vi "Handle Errors.vi"(8 "error in (no error)":errorcluster, 10 "Location":string, 11 "Mock Error Handler In":refnum<class "Mock Error Handler.lvclass">) -> (0 "error out":errorcluster, 3 "Mock Error Handler Out":refnum<class "Mock Error Handler.lvclass">)   [LabVIEW 2020, in "Mock Error Handler.lvclass"]
uses:
  Mock Error Handler.lvclass
  Mock Error Handler.lvclass/Mock Error Handler.ctl
  Private/Error Message Data.ctl
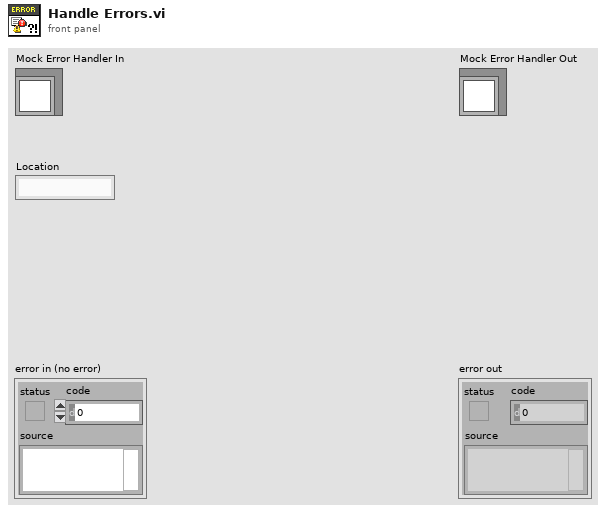
[diagram p1: front panel]
types:
  T1 = typedef "Mock Error Handler.lvclass/Error Message Data.ctl" = cluster{"Location":string, "Error":errorcluster}
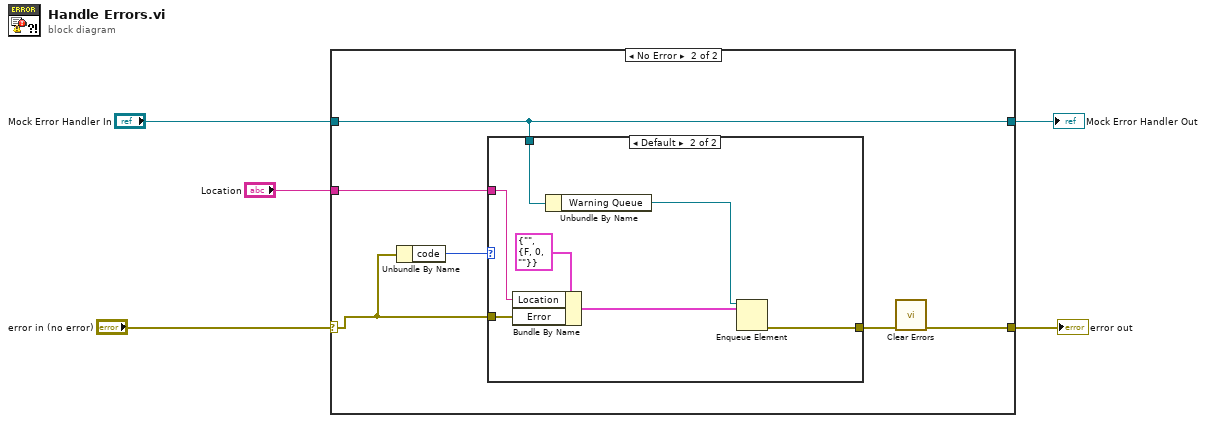
[diagram p0: block diagram]
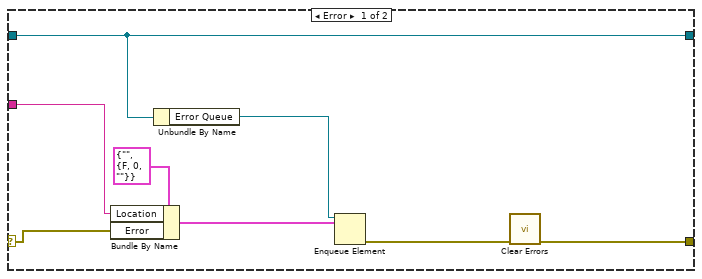
[diagram p2: hidden frame]
diagram:
  n1 = case shown="No Error" "error in (no error)" {
    selector: "error in (no error)" -> [w7 w15]
    tunnel: "Mock Error Handler In" -> [w13 w19]
    tunnel: [w13 w19] -> w5
    tunnel: [w6 w16] -> w1
    tunnel: "Location" -> [w8 w17]
    frame Error {
      n2 = Bundle By Name(cluster=T1 {"Location"="", "Error"={"status"=FALSE, "code"=0, "source"=""}} ("element"), "Location"=w8, "Error"=w7) -> (w9:T1)
      n3 = Unbundle By Name(w13) -> ("Error Queue"=w11:refnum<queue>)
      n4 = Enqueue Element(queue=w11, element=w9) -> (error out=w12:errorcluster)  [unwired: 2 in, 2 out]
      n5 = call <vilib>:"Clear Errors.vi"("error in (no error)"=w12) -> ("error out"=w6:errorcluster)  [unwired: 5 in, 1 out]
    }
    frame No Error {
      n6 = Unbundle By Name(w15) -> ("code"=w14:i32)
      n7 = case shown="Default" w14 {
        tunnel: w19 -> [_ w27]
        tunnel: [w20 w26] -> w18
        tunnel: w17 -> [_ w22]
        tunnel: w15 -> [w20 w21]
        frame 0 {
        }
        frame Default {
          n8 = Bundle By Name(cluster=T1 {"Location"="", "Error"={"status"=FALSE, "code"=0, "source"=""}} ("element"), "Location"=w22, "Error"=w21) -> (w23:T1)
          n9 = Unbundle By Name(w27) -> ("Warning Queue"=w25:refnum<queue>)
          n10 = Enqueue Element(queue=w25, element=w23) -> (error out=w26:errorcluster)  [unwired: 2 in, 2 out]
        }
      }
      n11 = call <vilib>:"Clear Errors.vi"("error in (no error)"=w18) -> ("error out"=w16:errorcluster)  [unwired: 5 in, 1 out]
    }
  }
  "error out" <- w1
  "Mock Error Handler Out" <- w5
